vi "Updating_day_files.vi"(5 "End time":timestamp, 6 "Start time":timestamp) -> ()   [LabVIEW 2010]
uses:
  Globals/Constants_global.vi
panel:
  out "Path name Out":path
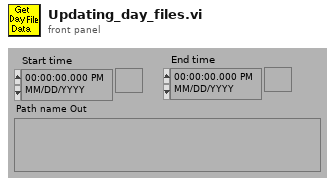
[diagram p1: front panel]
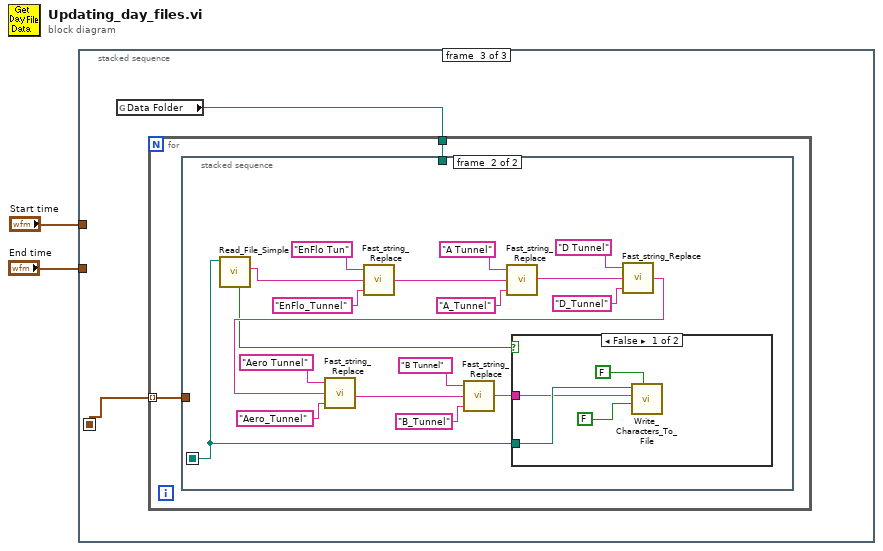
[diagram p0: block diagram]
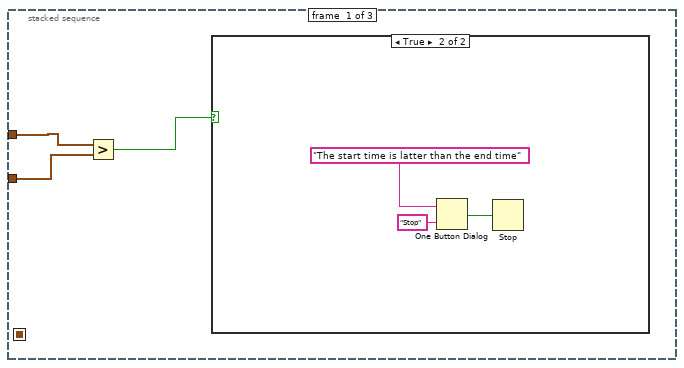
[diagram p2: hidden frame]
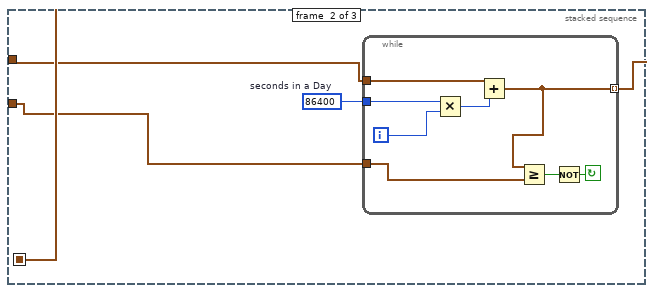
[diagram p4: hidden frame]
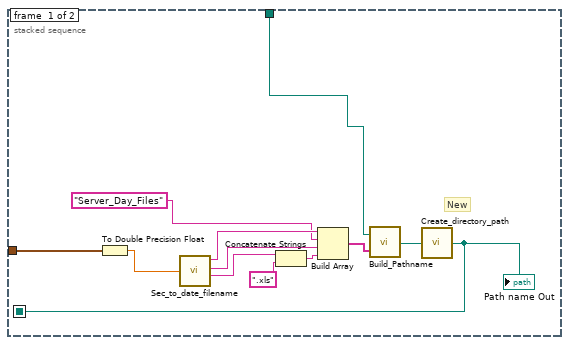
[diagram p5: hidden frame]
diagram:
  n1 = stacked-sequence {
    seq-local: [_ w12 _] -> [_ _ w22]
    tunnel: "End time" -> [w4 w9 _]
    tunnel: "Start time" -> [w3 w10 _]
    frame #0 {
      n2 = Greater?(x=w3, y=w4) -> (0:w5:bool)
      n3 = case shown="True" w5 {
        frame False {
        }
        frame True {
          n4 = One Button Dialog(message="The start time is latter than the end time", button name ("OK")="Stop") -> (true=w7:bool)
          n5 = Stop(stop? (T)=w7) -> ()
        }
      }
    }
    frame #1 {
      w11 = u32 86400  # seconds in a Day
      n6 = while {
        tunnel: [w13] -> w12 mode=indexing
        tunnel: w9 -> [w20]
        tunnel: w10 -> [w14]
        tunnel: w11 -> [w16]
        i -> [w17]
        stop <- w18 continue-if-true
        n7 = Multiply(x=w16, y=w17) -> (x*y=w15:u32)
        n8 = Add(x=w14, y=w15) -> (x+y=w13:timestamp)
        n9 = Greater Or Equal?(x=w13, y=w20) -> (x >= y?=w19:bool)
        n10 = Not(x=w19) -> (.not. x?=w18:bool)
      }
    }
    frame #2 {
      n11 = global read "Constants_global.vi" "Data Folder"() -> (w21:path)
      n12 = for {
        tunnel: w22 -> [w24] mode=indexing
        tunnel: w21 -> [w23]
        n13 = stacked-sequence {
          seq-local: [w25 _] -> [_ w38]
          tunnel: w24 -> [w36 _]
          tunnel: w23 -> [w26 _]
          frame #0 {
            # "New"
            n14 = To Double Precision Float(number=w36) -> (double precision float=w28:dbl)
            n15 = call "Sec_to_date_filename.vi"("seconds"=w28) -> ("Year"=w32:string, "Month"=w31:string, "Day"=w35:string)  [unwired: 1 out]
            n16 = Concatenate Strings(w35, ".xls" ("string")) -> (w33:string)
            n17 = Build Array(w32, "Server_Day_Files" ("Input Element"), w31, w33) -> (w29:string[])
            n18 = call "Build_Pathname.vi"("Output Array"=w29, "Pathname"=w26) -> ("Appended path"=w27:path)
            n19 = call "Create_directory_path.vi"("Path name"=w27) -> ("Path name Out"=w25:path)
            "Path name Out" <- w25
          }
          frame #1 {
            n20 = call "Read_File_Simple.vi"("Filename"=w38) -> ("Error?"=w39:bool, "string"=w54:string)  [unwired: 4 in, 4 out]
            n21 = call "Fast_string_Replace.vi"("Replace match with:"="EnFlo_Tunnel" ("regular expression"), "Input String"=w54, "regular expression"="EnFlo Tun") -> ("Output String"=w49:string)  [unwired: 1 in, 1 out]
            n22 = call "Fast_string_Replace.vi"("Replace match with:"="A_Tunnel" ("regular expression"), "Input String"=w49, "regular expression"="A Tunnel") -> ("Output String"=w46:string)  [unwired: 1 in, 1 out]
            n23 = call "Fast_string_Replace.vi"("Replace match with:"="D_Tunnel" ("regular expression"), "Input String"=w46, "regular expression"="D Tunnel") -> ("Output String"=w43:string)  [unwired: 1 in, 1 out]
            n24 = call "Fast_string_Replace.vi"("Replace match with:"="Aero_Tunnel" ("regular expression"), "Input String"=w43, "regular expression"="Aero Tunnel") -> ("Output String"=w40:string)  [unwired: 1 in, 1 out]
            n25 = call "Fast_string_Replace.vi"("Replace match with:"="B_Tunnel" ("regular expression"), "Input String"=w40, "regular expression"="B Tunnel") -> ("Output String"=w37:string)  [unwired: 1 in, 1 out]
            n26 = case shown="False" w39 {
              tunnel: w38 -> [w58 _]
              tunnel: w37 -> [w57 _]
              frame False {
                n27 = call "Write_Characters_To_File.vi"("file path (dialog if empty)"=w58, "advisory dialog? (display:T)"=FALSE, "character string"=w57, "append to file? (new file:F)"=FALSE) -> ()  [unwired: 4 in, 1 out]
              }
              frame True {
              }
            }
          }
        }
      }
    }
  }
